vi "CreatePizza.vi"(8 "error in (no error)":errorcluster, 11 "NYPizzaStore in":refnum<class "ChicagoPizzaStore.lvclass">) -> (0 "error out":errorcluster, 2 "YourPizzay":string, 3 "NYPizzaStore out":refnum<class "ChicagoPizzaStore.lvclass">)   [LabVIEW 2013, in "ChicagoPizzaStore.lvclass"]
uses:
  ChicagoPizzaStore.lvclass
  ChicagoPizzaIngredientFactory.lvclass/ChicagoPizzaIngredientFactory.lvclass
panel:
  # "我是芝加哥的比薩店"
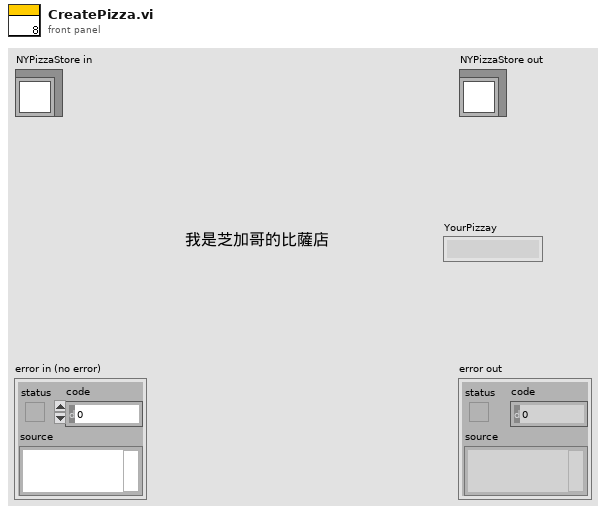
[diagram p1: front panel]
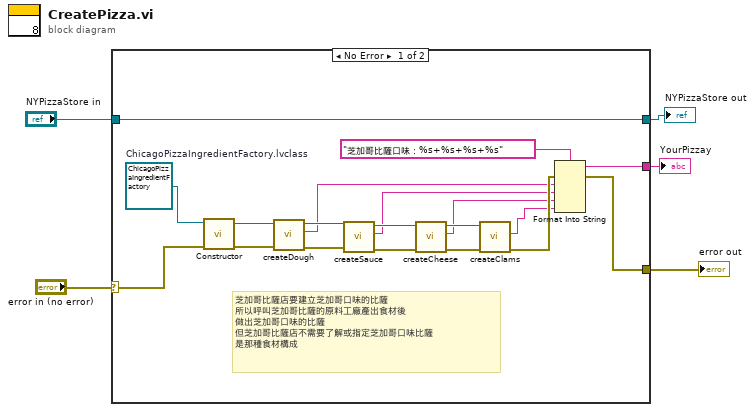
[diagram p0: block diagram]
diagram:
  n1 = case shown="No Error" "error in (no error)" {
    selector: "error in (no error)" -> [w16 w25]
    tunnel: [w15 w26] -> w4
    tunnel: "NYPizzaStore in" -> [w15 w26]
    tunnel: [w8 w25] -> w2
    tunnel: [w7 _] -> w1
    frame No Error {
      w6 = refnum<class "ChicagoPizzaIngredientFactory.lvclass"> refnum  # ChicagoPizzaIngredientFactory.lvclass
      # "芝加哥比薩店要建立芝加哥口味的比薩\n所以呼叫芝加哥比薩的原料工廠產出食材後\n做出芝加哥口味的比薩\n但芝加哥比薩店不需要了解或指定芝加哥口味比薩\n是那種食材構成"
      n2 = call-dynamic "Constructor.vi"("error in (no error)"=w16, "ChicagoPizzaIngredientFactory in"=w6) -> ("error out"=w20:errorcluster, "ChicagoPizzaIngredientFactory out"=w24:refnum<class "ChicagoPizzaIngredientFactory.lvclass">)  [unwired: 8 in]
      n3 = call-dynamic "createDough.vi"("error in (no error)"=w20, "ChicagoPizzaIngredientFactory in"=w24) -> ("error out"=w19:errorcluster, "Ingredients"=w12:string, "ChicagoPizzaIngredientFactory out"=w23:refnum<class "ChicagoPizzaIngredientFactory.lvclass">)  [unwired: 7 in]
      n4 = call-dynamic "createSauce.vi"("error in (no error)"=w19, "ChicagoPizzaIngredientFactory in"=w23) -> ("error out"=w18:errorcluster, "Ingredients"=w11:string, "ChicagoPizzaIngredientFactory out"=w22:refnum<class "ChicagoPizzaIngredientFactory.lvclass">)  [unwired: 7 in]
      n5 = call-dynamic "createCheese.vi"("error in (no error)"=w18, "ChicagoPizzaIngredientFactory in"=w22) -> ("error out"=w17:errorcluster, "Ingredients"=w10:string, "ChicagoPizzaIngredientFactory out"=w21:refnum<class "ChicagoPizzaIngredientFactory.lvclass">)  [unwired: 7 in]
      n6 = call-dynamic "createClams.vi"("error in (no error)"=w17, "ChicagoPizzaIngredientFactory in"=w21) -> ("error out"=w13:errorcluster, "Ingredients"=w9:string)  [unwired: 7 in, 1 out]
      n7 = Format Into String(format string="芝加哥比薩口味：%s+%s+%s+%s", error in=w13, w12, w11, w10, w9) -> (resulting string=w7:string, error out=w8:errorcluster)  [unwired: 1 in]
    }
    frame Error {
    }
  }
  "error out" <- w2
  "NYPizzaStore out" <- w4
  "YourPizzay" <- w1
